vi "SubVI_Set_47_arm.vi"(8 "error in (no error)":errorcluster, 11 "TCP Network Connection in":refnum<k5>) -> (0 "error out":errorcluster, 3 "TCP Network Connection out":refnum<k5>)   [LabVIEW 2020]
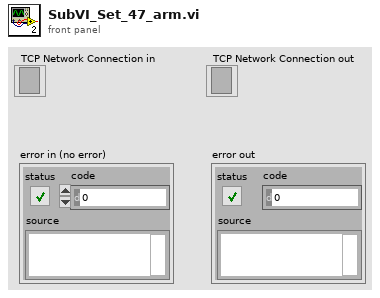
[diagram p1: front panel]
types:
  T1 = enum16{"Standard", "Buffered", "CRLF", "Immediate"}
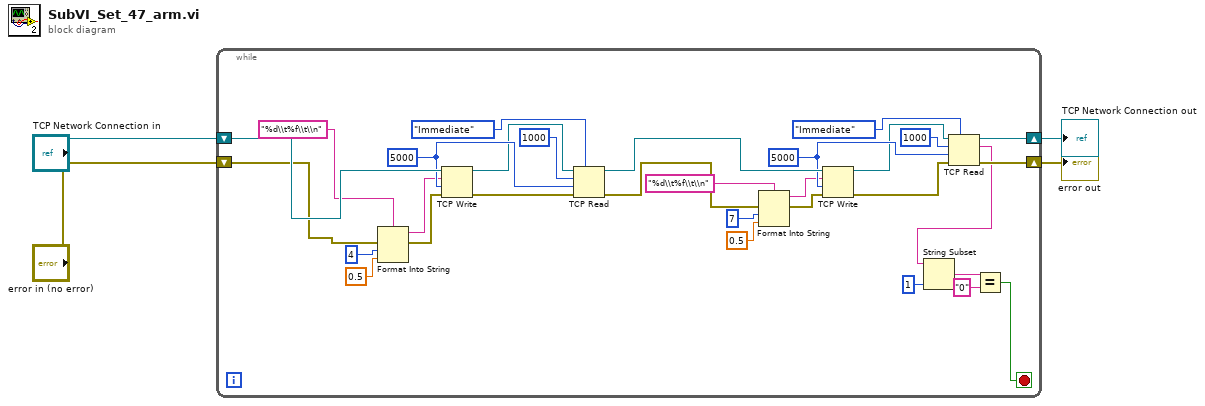
[diagram p0: block diagram]
diagram:
  n1 = while {
    shift-right: [w35] -> w4
    shift-left: "TCP Network Connection in" -> [w31]
    shift-right: [w34] -> w3
    shift-left: "error in (no error)" -> [w30]
    stop <- w5 stop-if-true
    w19 = 5000 ("timeout ms (25000)")
    w29 = 5000 ("timeout ms (25000)")
    n2 = Format Into String(format string="%d\\t%f\\t\\n", error in=w30, 4 ("input 1"), 0.5) -> (resulting string=w23:string, error out=w24:errorcluster)  [unwired: 1 in]
    n3 = TCP Write(connection ID=w31, data in=w23, error in (no error)=w24, 9:w29) -> (connection ID out=w26:refnum<k5>, error out=w25:errorcluster)  [unwired: 1 out]
    n4 = TCP Read(connection ID=w26, bytes to read=1000, error in (no error)=w25, 7:T1."Immediate" ("mode (standard)"), 9:w29) -> (connection ID out=w33:refnum<k5>, error out=w32:errorcluster)  [unwired: 1 out]
    n5 = Format Into String(format string="%d\\t%f\\t\\n", error in=w32, 7 ("input 1"), 0.5) -> (resulting string=w13:string, error out=w14:errorcluster)  [unwired: 1 in]
    n6 = TCP Write(connection ID=w33, data in=w13, error in (no error)=w14, 9:w19) -> (connection ID out=w16:refnum<k5>, error out=w15:errorcluster)  [unwired: 1 out]
    n7 = TCP Read(connection ID=w16, bytes to read=1000, error in (no error)=w15, 7:T1."Immediate" ("mode (standard)"), 9:w19) -> (connection ID out=w35:refnum<k5>, data out=w9:string, error out=w34:errorcluster)
    n8 = String Subset(string=w9, length (rest)=1 ("length (rest)")) -> (substring=w7:string)  [unwired: 1 in]
    n9 = Equal?(x=w7, y="0") -> (x = y?=w5:bool)
  }
  "TCP Network Connection out" <- w4
  "error out" <- w3
